vi "Load Config Application.vi"(8 "error In":errorcluster) -> (0 "error Out":errorcluster, 3 "Application Configuration":T1)   [LabVIEW 2021, in "Configuration.lvlib"]
uses:
  Configuration.lvlib
  Typedefs/Application Configuration.ctl
  Module Template/Typedefs/Config.ctl
  Core UI/Typedefs/Config.ctl
  Modules/Sound Manager/Typedefs/Config.ctl
  Utilities/Globales Snake.vi
  Module Template/Module Template.lvlib
  Core UI/Core UI.lvlib
  Modules/Sound Manager/Sound Manager.lvlib
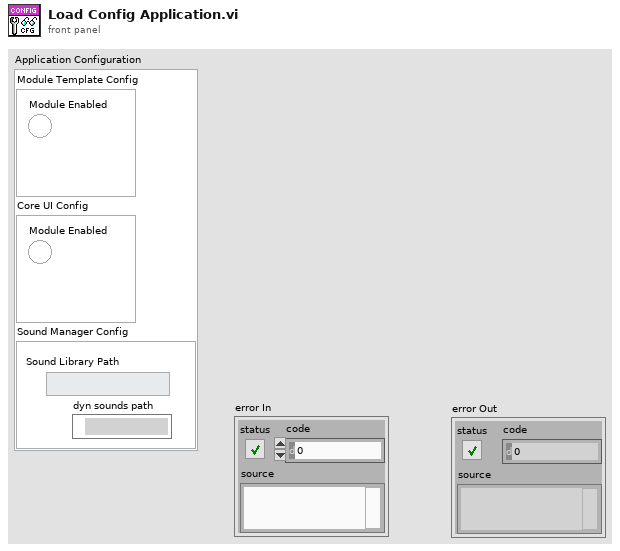
[diagram p1: front panel]
types:
  T1 = typedef "Configuration.lvlib/Application Configuration.ctl" = cluster{"Module Template Config":T2, "Core UI Config":T3, "Sound Manager Config":T4}
  T2 = typedef "Module Template.lvlib/Config.ctl" = cluster{"Module Enabled":bool}
  T3 = typedef "Core UI.lvlib/Config.ctl" = cluster{"Module Enabled":bool}
  T4 = typedef "Sound Manager.lvlib/Config.ctl" = cluster{"Sound Library Path":path, "dyn sounds path":path}
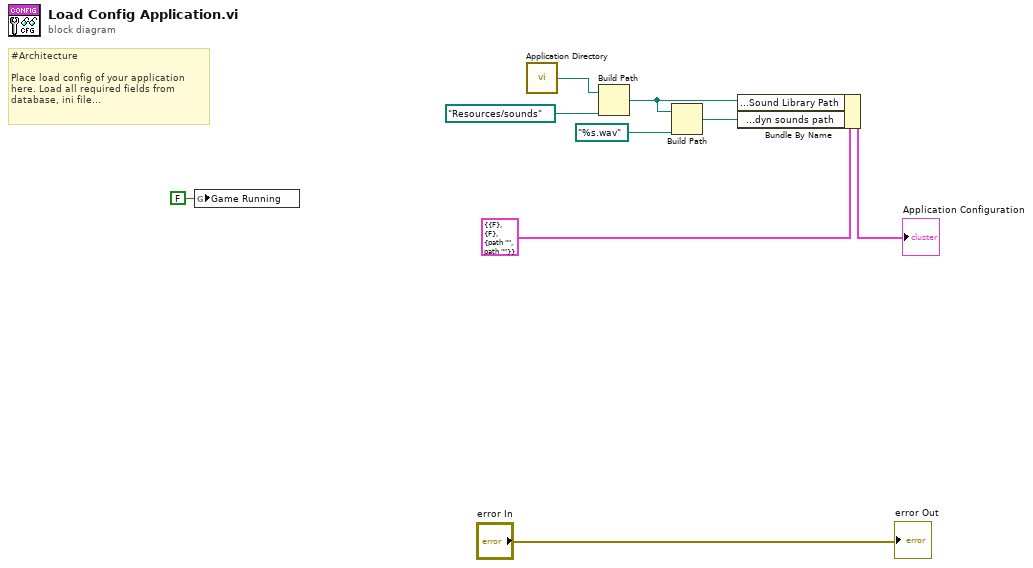
[diagram p0: block diagram]
diagram:
  # "#Architecture\n\nPlace load config of your application \nhere. Load all required fields from \ndatabase, ini file..."
  n1 = global write "Globales Snake.vi" "Game Running"(FALSE ("Game Running")) -> ()
  n2 = call <vilib>:"Application Directory.vi"() -> ("Application Directory"=w7:path)
  n3 = Build Path(base path=w7, name or relative path=path "Resources/sounds") -> (appended path=w3:path)
  n4 = Build Path(base path=w3, name or relative path=path "%s.wav") -> (appended path=w2:path)
  n5 = Bundle By Name(cluster=T1 {"Module Template Config"={"Module Enabled"=FALSE}, "Core UI Config"={"Module Enabled"=FALSE}, "Sound Manager Config"={"Sound Library Path"=path "", "dyn sounds path"=path ""}} ("Application Configuration"), "Sound Manager Config.Sound Library Path"=w3, "Sound Manager Config.dyn sounds path"=w2) -> (→"Application Configuration":T1)
  "error Out" <- "error In"
